vi "host_forTx_and_Rx_as scope.vi"() -> ()   [LabVIEW 2021]
uses:
  <vilib>/userdefined/High Color/nirio_resource_hc.ctl
  classes/5785_2_X_400MHz_Rx_as_scop/5785_2_X_400MHz_Rx_as_scop.lvclass
  CTL/user config.ctl
  CTL/emitter params.ctl
  CTL/mode_type.ctl
  <vilib>/Analysis/baseanly.llb/Mean (DBL).vi
  <vilib>/Utility/error.llb/Error Cluster From Error Code.vi
  <vilib>/rvi/errors/niLvFpgaAdjustHostInterfaceError.vi
  <instrlib>/FlexRIO/API/Host/v1/NI FlexRIO/API/Get Property Reference - Fpga Small.vi
  <instrlib>/_niInstr/Streaming/v1/Host/Public/Start Continuous Stream.vi
  <instrlib>/_niInstr/DSP/v1/FPGA/Public/Sub VIs/Data Conversion/U32 to IQ - 1 spc - S18.1.vi
  <vilib>/rvi/interface/nirviMethod/nirviMethod.xnode
  <vilib>/rvi/interface/nirviReadWriteControl/nirviReadWriteControl.xnode
  <vilib>/FPGAPlugInAG/Dynamic/niLvFpga_ReadFifo_Dynamic.vi
  <vilib>/rvi/errors/niLvFpgaMergeErrorWithErrorCode.vi
  <instrlib>/_niInstr/DSP/v1/FPGA/niInstr DSP v1 FPGA.lvlib
  <vilib>/Analysis/NI_AALBase.lvlib
  NiFpgaLv.dll
  <vilib>/rvi/interface/Simulation/niFpgaSimulationCallBeginRW.vi
  <instrlib>/_niInstr/Streaming/v1/Host/niInstr Streaming v1 Host.lvlib
  <resource>/objmgr/niflexrioapi.rc
  <instrlib>/FlexRIO/API/Host/v1/NI FlexRIO API v1.lvlib
panel:
  out "delta time over time":dbl[][](graph)
  out "delta time":dbl[](array[numeric])=[-3.384901075355306e-11] format="%#_6p"
  in  "Tab Control":T1(tab)=enum."Rx set up"
  in  "devicess":T2[](array[typedef])=["IF_transceiver_0", "IF_transceiver_1", "IF_transceiver_2"]
  in  "frequency list":dbl[](array[numeric])=[120000000.0, 250000000.0, 50000000.0, 200000000.0, 100000000.0, 300000000.0, 160000000.0, 220000000.0, 150000000.0] format="%#_6pHz"
  in  "d phase 2":dbl=1e-06
  in  "threshold":dbl=-60.0 format="%0.2f"
  in  "number of sampels per test":u32=10000
  in  "reciever num":i32=2
  in  "one device":bool=TRUE
  out "dt":dbl[](array[numeric]) format="%#_6p"
  out "dt mean":dbl[](array[numeric]) format="%#_6p"
  in  "time calibrate":dbl[](array[numeric])=[2.34863e-10, -9.70626e-11, 0.0] format="%#_6p"
  out "phase DAC Value":i32[](array[numeric])=[1000, 1387, 1016]
  out "d phase":cluster{"frequncy":dbl[], "d phase":dbl[]}[](graph)=[{"frequncy"=[50003786.05147211, 99994198.20913488, 120000208.59128165, 150004249.47974658, 159998464.34553584, 199999299.07078186, 219990729.91948402, 250003148.13745588, 300002773.74392134], "d phase"=[-0.3585033135275353, -0.8011119407067326, -1.6642934286416562, -2.38221684538712, -2.2648984836965838, -2.180939515591376, -2.521274049342594, -3.7939032623280013, -3.912898695939134]}]
  out "spectrum":cluster{"f0":dbl, "df":dbl, "magnitude":dbl[]}[](graph)=[{"f0"=-50000000.0, "df"=40000.0, "magnitude"=array[10000 elements]}, {"f0"=-50000000.0, "df"=40000.0, "magnitude"=array[10000 elements]}]
  in  "Stop":bool
  out "scope":dbl[][](graph)
  out "dds free":bool[][](array[boolean])=[[FALSE, FALSE, FALSE, FALSE, FALSE, FALSE], [FALSE, FALSE, FALSE, FALSE, FALSE, FALSE], [FALSE, FALSE, FALSE, FALSE, FALSE, FALSE], [FALSE, FALSE, FALSE, FALSE, FALSE, FALSE], [FALSE, FALSE, FALSE, FALSE, FALSE, FALSE], [FALSE, FALSE, FALSE, FALSE, FALSE, FALSE], [FALSE, FALSE, FALSE, FALSE, FALSE, FALSE], [FALSE, FALSE, FALSE, FALSE, FALSE, FALSE], [FALSE, FALSE, FALSE, FALSE, FALSE, FALSE], [TRUE, TRUE, TRUE, TRUE, TRUE, TRUE], [TRUE, TRUE, TRUE, TRUE, TRUE, TRUE], [TRUE, TRUE, TRUE, TRUE, TRUE, TRUE], [TRUE, TRUE, TRUE, TRUE, TRUE, TRUE], [TRUE, TRUE, TRUE, TRUE, TRUE, TRUE], [TRUE, TRUE, TRUE, TRUE, TRUE, TRUE], [TRUE, TRUE, TRUE, TRUE, TRUE, TRUE]]
  out "secnario elapest":dbl=738.0
  # "Tx state"
  # "Rx state"
  # "for zero put epsilon (almost zero)"
  # "1-2\n2-3\n3-1"
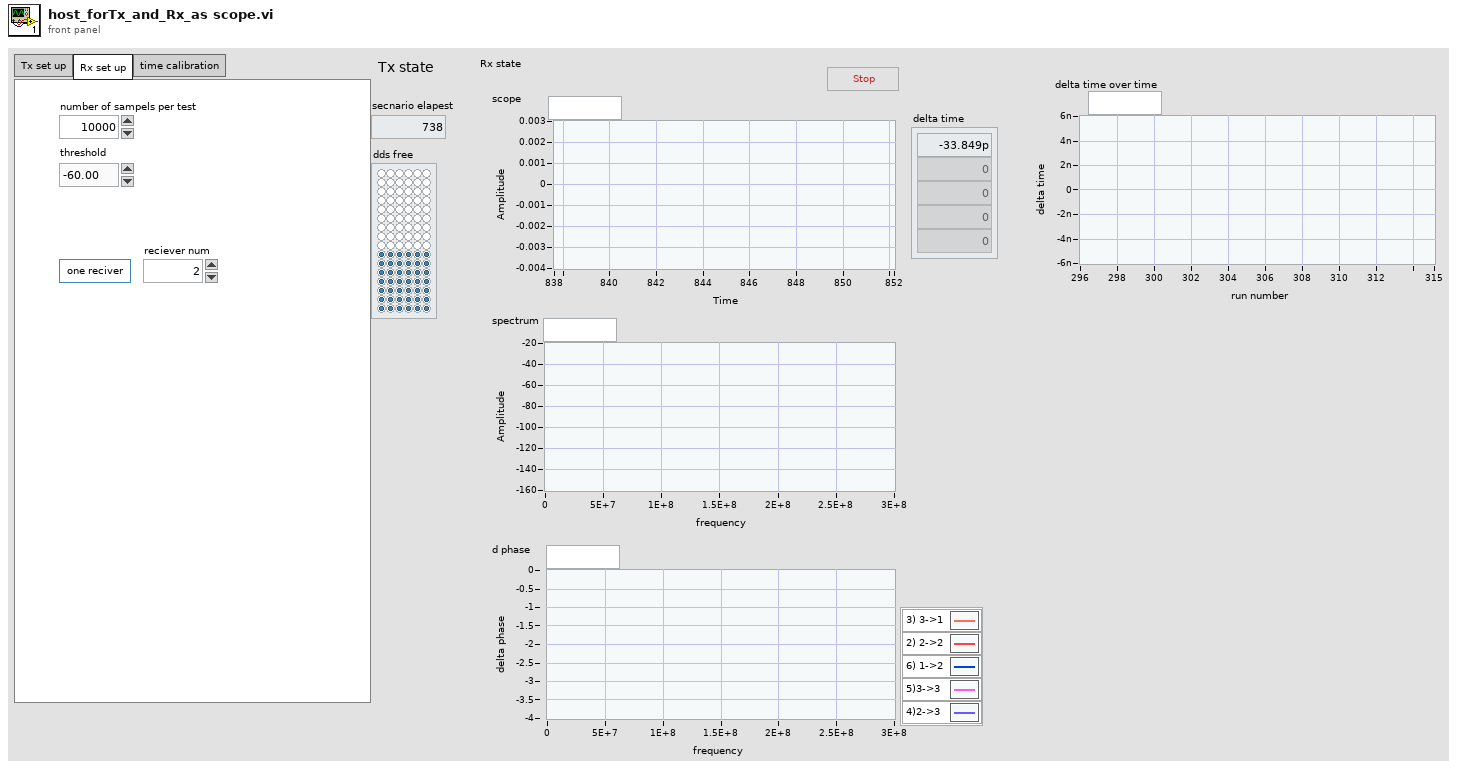
[diagram p1: front panel]
types:
  T1 = enum32{"Tx set up", "Rx set up", "time calibration"}
  T2 = typedef "nirio_resource_hc.ctl" = tag
  T3 = typedef "user config.ctl" = cluster{"vst_device":refnum<k15>[], "RF gain ":dbl, "buffer size":u32, "center frequency (Hz) ":dbl, "P2P sample rate":dbl, "mode":enum16{"USRP - 180MHz", "5785 - 2*180MHz", "5785 - 3.2GHz", "P2P - VST"}, "devicess":T2[], "gen for df":bool, "Rx settings":cluster{"min PW         ":dbl, "max gap        ":dbl, "detection bar":dbl, "peak detect                        ":bool}, "use arb files":bool}
  T4 = typedef "mode_type.ctl" = enum8{"CW", "from memory 1", "NC - cw", "LFM", "BPSK", "QPSK"}
  T5 = typedef "emitter params.ctl" = cluster{"f set":dbl[], "hop rate (Hz)":dbl, "d.c.":dbl, "amp (dB)":dbl, "mod type":T4, "mod depth":dbl, "DOA":dbl, "t start":dbl, "t end":dbl}
  T6 = typedef "PDW_lv2.ctl" = cluster{"t start":dbl, "frequency (Hz)":dbl, "duration (sec)":dbl, "amp (lin)":dbl, "mod type":T4, "mod depth":dbl, "phase (rad)":dbl[]}
  T7 = cluster{"fpga clock":dbl, "pulse transmitted":u32, "dds free":bool[][]}
  T8 = typedef "niInstr DSP v1 Shared.lvlib/IQ Data.ctl" = cluster{"I":fxp<+/-,18,1>, "Q":fxp<+/-,18,1>, "overflow":bool}
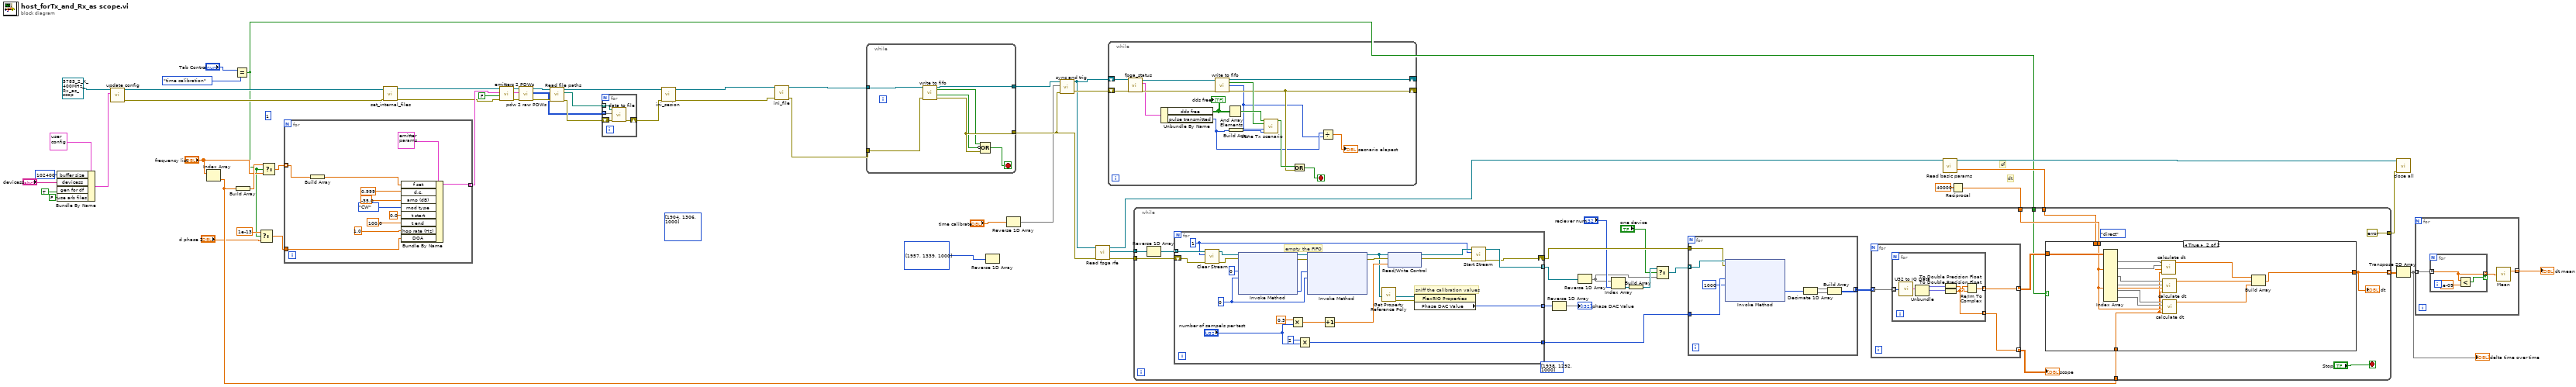
[diagram p0: block diagram]
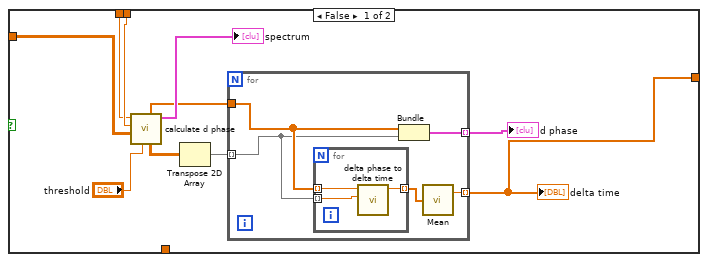
[diagram p2: hidden frame]
diagram:
  (unwired) i32[] [1904, 1306, 1000] ("Array")
  (unwired) 1
  # "cf"
  # "dt"
  n1 = Bundle By Name(cluster=T3 {"vst_device"=["VST_1", "VST_2"], "RF gain "=10.0, "buffer size"=524288, "center frequency (Hz) "=1000000000.0, "P2P sample rate"=200000000.0, "mode"=enum."5785 - 2*180MHz", "devicess"=["IF_transiver_0", "IF_transiver_1", "IF_transiver_2"], "gen for df"=FALSE, "Rx settings"={"min PW         "=0.0, "max gap        "=0.0, "detection bar"=0.0, "peak detect                        "=FALSE}, "use arb files"=TRUE} ("user configurations"), "buffer size"=u32 102400, "devicess"="devicess", "gen for df"=TRUE, "use arb files"=FALSE) -> (w2:T3)
  n2 = call-dynamic "update config.vi"("user configurations"=w2, "5785_2_X_400MHz_Rx_as_scop in"=refnum<class "5785_2_X_400MHz_Rx_as_scop.lvclass"> refnum ("5785_2_X_400MHz_Rx_as_scop.lvclass")) -> ("error out"=w52:errorcluster, "5785_2_X_400MHz_Rx_as_scop out"=w22:refnum<class "5785_2_X_400MHz_Rx_as_scop.lvclass">)  [unwired: 6 in, 2 out]
  n3 = Index Array(array="frequency list") -> (element=w15:dbl)  [unwired: 1 in]
  n4 = Equal?(x="Tab Control", y=T1."time calibration") -> (x = y?=w6:bool)
  n5 = Build Array(w15) -> (w13:dbl[])
  n6 = Select(t=1e-13, s=w6, f="d phase 2") -> (s? t:f=w8:dbl)
  n7 = Select(t=w13, s=w6, f="frequency list") -> (s? t:f=w16:dbl[])
  n8 = for {
    tunnel: [w65] -> w43 mode=indexing
    tunnel: w16 -> [w57] mode=indexing
    tunnel: w8 -> [w56]
    n9 = Build Array(w57) -> (w66:dbl[])
    n10 = Bundle By Name(cluster=T5 {"f set"=[], "hop rate (Hz)"=0.0, "d.c."=0.0, "amp (dB)"=0.0, "mod type"=enum."CW", "mod depth"=0.0, "DOA"=0.0, "t start"=0.0, "t end"=0.0} ("Cluster"), "f set"=w66, "d.c."=0.999, "amp (dB)"=-35.0, "mod type"=mode_type."CW", "t start"=0.0, "t end"=100.0, "hop rate (Hz)"=1.0, "DOA"=w56) -> (w65:T5)
  }
  n11 = call-dynamic "set_internal_files.vi"("error in (no error)"=w52, "device_type in"=w22) -> ("error out"=w36:errorcluster, "device_type out"=w37:refnum<class "5785_2_X_400MHz_Rx_as_scop.lvclass">)  [unwired: 8 in]
  n12 = call-dynamic "emitters 2 PDWs.vi"("error in (no error)"=w36, "random startinig phase"=FALSE, "emmiter"=w43, "device_type in"=w37) -> ("error out"=w42:errorcluster, "sorted PDWs"=w41:T6[], "device_type out"=w40:refnum<class "5785_2_X_400MHz_Rx_as_scop.lvclass">)  [unwired: 5 in]
  n13 = call-dynamic "pdw 2 raw PDWs.vi"("error in (no error)"=w42, "PDWs"=w41, "device_type in"=w40) -> ("error out"=w38:errorcluster, "Array"=w23:u64[][], "device_type out"=w34:refnum<class "5785_2_X_400MHz_Rx_as_scop.lvclass">)  [unwired: 6 in]
  n14 = call-dynamic "Read file paths.vi"("error in (no error)"=w38, "device_type in"=w34) -> ("error out"=w35:errorcluster, "file paths"=w24:path[], "device_type out"=w33:refnum<class "5785_2_X_400MHz_Rx_as_scop.lvclass">)  [unwired: 6 in, 1 out]
  n15 = for {
    tunnel: w23 -> [w68] mode=indexing
    shift-right: [w69] -> w32
    shift-left: w35 -> [w70]
    tunnel: w24 -> [w67] mode=indexing
    n16 = call "data to file.vi"("error in (no error)"=w70, "Array"=w68, "Path"=w67) -> ("error out"=w69:errorcluster)  [unwired: 8 in]
  }
  n17 = call-dynamic "ini_sesion.vi"("error in (no error)"=w32, "5785_2_X_400MHz_Rx_as_scop in"=w33) -> ("error out"=w53:errorcluster, "5785_2_X_400MHz_Rx_as_scop out"=w54:refnum<class "5785_2_X_400MHz_Rx_as_scop.lvclass">)  [unwired: 8 in]
  n18 = call-dynamic "ini_file.vi"("device_type in"=w54, "error in (no error)"=w53) -> ("device_type out"=w51:refnum<class "5785_2_X_400MHz_Rx_as_scop.lvclass">, "error out"=w50:errorcluster)  [unwired: 11 in, 1 out]
  n19 = while {
    tunnel: w51 -> [w77]
    tunnel: w50 -> [w76]
    tunnel: [w75] -> w49
    tunnel: [w73] -> w30
    stop <- w74 stop-if-true
    n20 = call-dynamic "write to fifo.vi"("5785_2_X_400MHz_Rx_as_scop in"=w77, "error in (no error)"=w76) -> ("5785_2_X_400MHz_Rx_as_scop out"=w75:refnum<class "5785_2_X_400MHz_Rx_as_scop.lvclass">, "done write file"=w71:bool, "room on fifo"=w72:bool, "error out"=w73:errorcluster)  [unwired: 9 in, 1 out]
    n21 = Compound Arithmetic op=OR(w71, invert w72, w73) -> (w74:bool)
  }
  n22 = Reverse 1D Array(array=i32[] [1957, 1339, 1000] ("Array")) -> ()  [unwired: 1 out]
  n23 = Reverse 1D Array(array="time calibrate") -> (reversed array=w4:dbl[])
  n24 = call-dynamic "sync and trig.vi"("error in (no error)"=w30, "time calibrate"=w4, "5785_2_X_400MHz_Rx_as_scop in"=w49) -> ("error out"=w48:errorcluster, "5785_2_X_400MHz_Rx_as_scop out"=w31:refnum<class "5785_2_X_400MHz_Rx_as_scop.lvclass">)  [unwired: 7 in]
  n25 = call-dynamic "Read fpga rfe.vi"("error in (no error)"=w30, "5785_2_X_400MHz_Rx_as_scop in"=w31) -> ("error out"=w29:errorcluster, "fpga rfe"=w28:refnum<k20>[], "5785_2_X_400MHz_Rx_as_scop out"=w21:refnum<class "5785_2_X_400MHz_Rx_as_scop.lvclass">)  [unwired: 6 in, 1 out]
  n26 = while {
    shift-right: [w89] -> _
    shift-left: w31 -> [w91]
    shift-right: [w82] -> _
    shift-left: w48 -> [w90]
    stop <- w81 stop-if-true
    n27 = call-dynamic "fpga_status.vi"("error in (no error)"=w90, "5785_2_X_400MHz_Rx_as_scop in"=w91) -> ("error out"=w92:errorcluster, "pulse TX status"=w87:T7, "5785_2_X_400MHz_Rx_as_scop out"=w93:refnum<class "5785_2_X_400MHz_Rx_as_scop.lvclass">)  [unwired: 7 in]
    n28 = Unbundle By Name(w87) -> ("dds free"=w86:bool[][], "pulse transmitted"=w80:u32)
    "dds free" <- w86
    n29 = call-dynamic "write to fifo.vi"("5785_2_X_400MHz_Rx_as_scop in"=w93, "error in (no error)"=w92) -> ("5785_2_X_400MHz_Rx_as_scop out"=w89:refnum<class "5785_2_X_400MHz_Rx_as_scop.lvclass">, "done write file"=w85:bool, "num of pulses sent to the FPGA"=w79:u32, "error out"=w82:errorcluster)  [unwired: 9 in, 1 out]
    n30 = And Array Elements(Boolean array=w86) -> (logical AND=w88:bool)
    n31 = Build Array(w80) -> (w84:u32[])
    n32 = call "done Tx scenario.vi"("all dds free"=w88, "done write files"=w85, "num of pulse sent to fpga"=w79, "pulse transmitted"=w84) -> ("Done Tx secenario?"=w83:bool)  [unwired: 11 in]
    n33 = Or(x=w83, y=w82) -> (x .or. y?=w81:bool)
    n34 = Divide(x=w80, y=w79) -> (x/y=→"secnario elapest":dbl)
  }
  n35 = call-dynamic "Read basic params.vi"("device_type in"=w21) -> ("device_type out"=w20:refnum<class "5785_2_X_400MHz_Rx_as_scop.lvclass">, "center frequency (Hz)"=w19:dbl)  [unwired: 12 in, 5 out]
  n36 = Reciprocal(x=400000000.0) -> (1/x=w26:dbl)
  n37 = while {
    tunnel: w29 -> [w112]
    tunnel: w28 -> [w111]
    tunnel: w26 -> [w101]
    tunnel: [errorcluster {"status"=FALSE, "code"=0, "source"=""} ("error out")] -> w25
    tunnel: w19 -> [w99]
    tunnel: w15 -> [w100]
    tunnel: [w102] -> w18 mode=indexing
    tunnel: w6 -> [w96]
    stop <- "Stop" stop-if-true
    (unwired) i32[] [1938, 1292, 1000] ("Array")
    (unwired) enum32{"direct", "frequency domain"}."direct" ("algorithm")
    n38 = Reverse 1D Array(array=w111) -> (reversed array=w110:refnum<k20>[])
    n39 = for {
      tunnel: w110 -> [w166] mode=indexing
      tunnel: [w159] -> w98 mode=indexing
      tunnel: [w167] -> w114
      shift-right: [w158] -> w113
      shift-left: w112 -> [w165]
      tunnel: [w152] -> w95 mode=indexing
      w149 = 0 ("Timeout (ms)")
      w161 = 1 ("stream index")
      # "sniff the calibration values"
      # "empty the FIFO"
      n40 = call <instrlib>:"Clear Stream.vi"("error in (no error)"=w165, "stream index"=w161, "refnum in"=w166) -> ("error out"=w163:errorcluster, "refnum out"=w164:refnum<k20>)  [unwired: 7 in]
      n41 = xnode "Invoke Method"("FPGA VI Reference In"=w164, "error in"=w163, "Number of Elements"=u32 0, "Timeout (ms)"=w149) -> ("FPGA VI Reference Out"=w171:refnum<k20>, "error out"=w172:errorcluster, "Elements Remaining"=w151:u32)  [unwired: 1 out]
      n42 = Multiply(x=0.5, y="number of sampels per test") -> (x*y=w157:dbl)
      n43 = Multiply(x=u32 2, y="number of sampels per test") -> (x*y=w167:u32)
      n44 = xnode "Invoke Method"("FPGA VI Reference In"=w171, "error in"=w172, "Number of Elements"=w151, "Timeout (ms)"=w149) -> ("FPGA VI Reference Out"=w155:refnum<k20>, "error out"=w170:errorcluster)  [unwired: 2 out]
      n45 = Increment(x=w157) -> (x+1=w156:dbl)
      n46 = call-poly <instrlib>:"Get Property Reference Poly.vi"("fpga interface in"=w155) -> ("error out"=w153:errorcluster, "property reference"=w154:refnum<k20>)  [unwired: 5 in, 1 out]
      n47 = xnode "Read/Write Control"("FPGA VI Reference In"=w155, "error in"=w170, "rx count .5"=w156) -> ("FPGA VI Reference Out"=w162:refnum<k20>, "error out"=w160:errorcluster)
      n48 = property class="FlexRIO Properties"(reference=w154, error in=w153) -> ("Phase DAC Value"=w152:i32)  [unwired: 2 out]
      n49 = call-poly <instrlib>:"Start Stream.vi"("error in (no error)"=w160, "stream index"=w161, "refnum in"=w162) -> ("error out"=w158:errorcluster, "refnum out"=w159:refnum<k20>)  [unwired: 7 in]
    }
    n50 = Reverse 1D Array(array=w95) -> (reversed array=→"phase DAC Value":i32[])
    n51 = Reverse 1D Array(array=w98) -> (reversed array=w97:refnum<k20>[])
    n52 = Index Array(array=w97, index="reciever num") -> (element=w109:refnum<k20>)
    n53 = Build Array(w109) -> (w107:refnum<k20>[])
    n54 = Select(t=w107, s="one device", f=w97) -> (s? t:f=w105:refnum<k20>[])
    n55 = for {
      tunnel: w105 -> [w180] mode=indexing
      tunnel: [w181] -> w116 mode=concatenating
      tunnel: w114 -> [w179]
      tunnel: w113 -> [w176]
      n56 = xnode "Invoke Method"("FPGA VI Reference In"=w180, "error in"=w176, "Number of Elements"=w179, "Timeout (ms)"=1000) -> ("Data"=w177:u32[])  [unwired: 3 out]
      n57 = Decimate 1D Array(w177) -> (w175:u32[], w174:u32[])
      n58 = Build Array(w175, w174) -> (w181:u32[][])
    }
    n59 = for {
      tunnel: w116 -> [w184] mode=indexing
      tunnel: [w183] -> w103 mode=indexing
      tunnel: [w182] -> w115 mode=indexing
      n60 = for {
        tunnel: w184 -> [w191] mode=indexing
        tunnel: [w188] -> w183 mode=indexing
        tunnel: [w185] -> w182 mode=indexing
        n61 = call-poly <instrlib>:"U32 to IQ Data.vi"("U32 data"=w191) -> ("IQ data"=w190:T8)  [unwired: 14 in]
        n62 = Unbundle(w190) -> ("I"=w187:fxp<+/-,18,1>, "Q"=w189:fxp<+/-,18,1>)  [unwired: 1 out]
        n63 = To Double Precision Float(number=w187) -> (double precision float=w186:dbl)
        n64 = To Double Precision Float(number=w189) -> (double precision float=w185:dbl)
        n65 = Re/Im To Complex(1:w186, 2:w185) -> (0:w188:cdb)
      }
    }
    "scope" <- w115
    n66 = case shown="True" w96 {
      tunnel: w103 -> [w127 w148]
      tunnel: [w118 w142] -> w102
      tunnel: w101 -> [w126 w137]
      tunnel: w100 -> [_ w136]
      tunnel: w99 -> [w125 _]
      frame False {
        n67 = call "calculate d phase.vi"("threshold"="threshold", "IQ in"=w127, "dt"=w126, "center frequency (Hz)"=w125) -> ("spectrum"=→"spectrum":cluster{"f0":dbl, "df":dbl, "magnitude":dbl[]}[], "d phase"=w120:dbl[][], "frequncy"=w122:dbl[])  [unwired: 3 in, 2 out]
        n68 = Transpose 2D Array(2D array=w120) -> (transposed array=w119:dbl[][])
        n69 = for {
          tunnel: w119 -> [w130] mode=indexing
          tunnel: w122 -> [w131]
          tunnel: [w132] -> w121 mode=indexing
          tunnel: [w128] -> w118 mode=indexing
          n70 = for {
            tunnel: w131 -> [w135] mode=indexing
            tunnel: w130 -> [w134] mode=indexing
            tunnel: [w133] -> w129 mode=indexing
            n71 = call "delta phase to delta time.vi"("delta phase (deg)"=w134, "freqency"=w135) -> ("delta time"=w133:dbl)  [unwired: 9 in]
          }
          n72 = Bundle("frequncy"=w131, w130) -> (w132:cluster{"frequncy":dbl[], dbl[]})  [unwired: 1 in]
          n73 = call-poly <vilib>:"Mean.vi"("X"=w129) -> ("mean"=w128:dbl)  [unwired: 1 out]
        }
        "d phase" <- w121
        "delta time" <- w118
      }
      frame True {
        n74 = Index Array(array=w148) -> (element #1=w139:cdb[], element #2=w141:cdb[], element #3=w140:cdb[], element #4=w147:cdb[], element #5=w138:cdb[], element #6=w146:cdb[])  [unwired: 12 in]
        n75 = call "calculate dt.vi"("f test"=w136, "dt sampels"=w137, "Array 2"=w141, "Array"=w139) -> ("d t stream"=w145:dbl)  [unwired: 7 in]
        n76 = call "calculate dt.vi"("f test"=w136, "dt sampels"=w137, "Array 2"=w147, "Array"=w140) -> ("d t stream"=w144:dbl)  [unwired: 7 in]
        n77 = call "calculate dt.vi"("f test"=w136, "dt sampels"=w137, "Array 2"=w146, "Array"=w138) -> ("d t stream"=w143:dbl)  [unwired: 7 in]
        n78 = Build Array(w145, w144, w143) -> (w142:dbl[])
      }
    }
    "dt" <- w102
  }
  n79 = Transpose 2D Array(2D array=w18) -> (transposed array=w3:dbl[][])
  "delta time over time" <- w3
  n80 = call-dynamic "close all.vi"("error in (no error)"=w25, "5785_2_X_400MHz_Rx_as_scop in"=w20) -> ()  [unwired: 8 in, 2 out]
  n81 = for {
    tunnel: [w194] -> w17 mode=indexing
    tunnel: w3 -> [w193] mode=indexing
    n82 = for {
      tunnel: w193 -> [w196] mode=indexing
      tunnel: [w196] -> w192 mode=indexing if=w195
      n83 = Less?(x=w196, y=1e-09) -> (x < y?=w195:bool)
    }
    n84 = call-poly <vilib>:"Mean.vi"("X"=w192) -> ("mean"=w194:dbl)  [unwired: 1 out]
  }
  "dt mean" <- w17
